vi "GearGroup.vi"(6 "Line Border":cluster{"Top":dbl, "Bottom":dbl}={"Top"=6.0, "Bottom"=1.0}, 8 "Padding for Rectangle":dbl=5.0 format="%#_13g", 9 "Score Cutoff":dbl=3.0, 10 "Sorted Data":dbl[][](array[numeric])) -> (0 "Rect":T1, 1 "Line":T1, 2 "Score":dbl, 3 "Center":cluster{"X":dbl, "Y":dbl})   [LabVIEW 2016]
panel:
  out "Grouping Scores":T2(array[cluster])
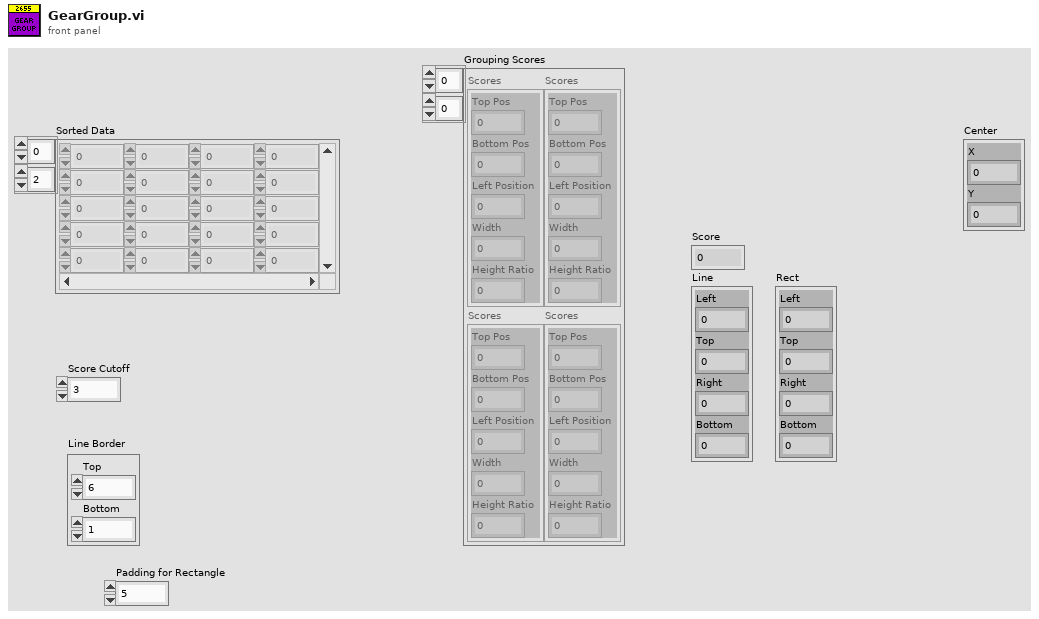
[diagram p1: front panel]
types:
  T1 = cluster{"Left":dbl, "Top":dbl, "Right":dbl, "Bottom":dbl}
  T2 = cluster{"Top Pos":dbl, "Bottom Pos":dbl, "Left Position":dbl, "Width":dbl, "Height Ratio":dbl}[][]
  T3 = cluster{"Top Position":dbl, "Bottom Position":dbl, "Top Gap":dbl, "Width":dbl, "Height Ratio":dbl}
  T4 = cluster{"Left":dbl, "Numeric":dbl, "Right":dbl, "Numeric":dbl}
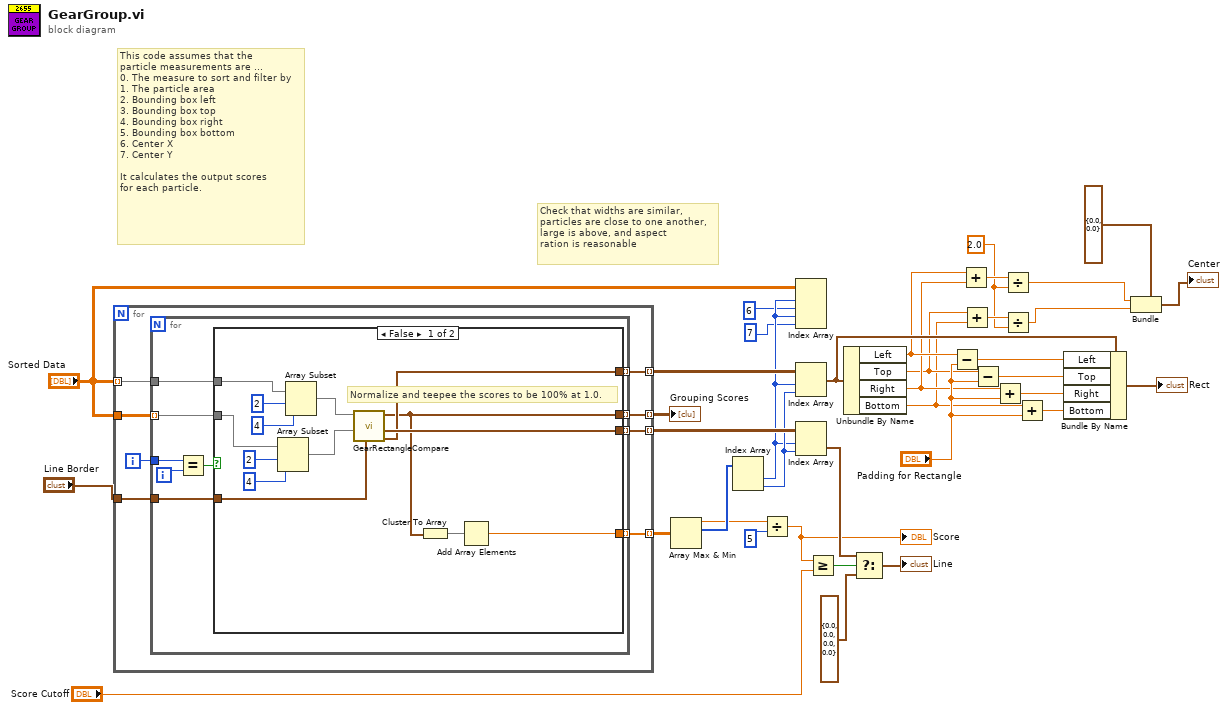
[diagram p0: block diagram]
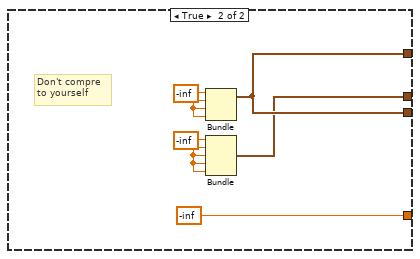
[diagram p2: hidden frame]
diagram:
  w3 = 2.0 ("y")
  # "Check that widths are similar,\nparticles are close to one another,\nlarge is above, and aspect\nration is reasonable"
  # "This code assumes that the\nparticle measurements are ...\n0. The measure to sort and filter by\n1. The particle area\n2. Bounding box left\n3. Bounding box top\n4. Bounding box right\n5. Bounding box bottom\n6. Center X\n7. Center Y\n\nIt calculates the output scores\nfor each particle."
  n1 = for {
    tunnel: "Sorted Data" -> [w45] mode=indexing
    tunnel: "Sorted Data" -> [w44]
    tunnel: [w43] -> w37 mode=indexing
    tunnel: [w41] -> w36 mode=indexing
    tunnel: [w40] -> w33 mode=indexing
    tunnel: [w39] -> w29 mode=indexing
    tunnel: "Line Border" -> [w38]
    i -> [w42]
    n2 = for {
      tunnel: w45 -> [w55]
      tunnel: w44 -> [w53] mode=indexing
      tunnel: [w52] -> w43 mode=indexing
      tunnel: w42 -> [w51]
      tunnel: [w49] -> w41 mode=indexing
      tunnel: [w48] -> w40 mode=indexing
      tunnel: [w47] -> w39 mode=indexing
      tunnel: w38 -> [w46]
      i -> [w50]
      n3 = Equal?(x=w51, y=w50) -> (x = y?=w54:bool)
      n4 = case shown="False" w54 {
        tunnel: w55 -> [w67 _]
        tunnel: w53 -> [w64 _]
        tunnel: [w58 w70] -> w52
        tunnel: [w62 -inf] -> w49
        tunnel: [w60 w73] -> w48
        tunnel: [w59 w73] -> w47
        tunnel: w46 -> [w56 _]
        frame False {
          # "Normalize and teepee the scores to be 100% at 1.0."
          n5 = Array Subset(array=w64, index=2, length=4) -> (w61:dbl[])
          n6 = Array Subset(array=w67, index=2, length=4) -> (w57:dbl[])
          n7 = call "GearRectangleCompare.vi"("Line Border"=w56, "Second"=w61, "First"=w57) -> ("Rect"=w59:T1, "Line"=w60:T1, "Scores"=w58:T3)  [unwired: 6 in]
          n8 = Cluster To Array(cluster=w58) -> (array=w63:dbl[])
          n9 = Add Array Elements(numeric array=w63) -> (sum=w62:dbl)
        }
        frame True {
          w71 = -inf
          w72 = -inf
          # "Don't compre\nto yourself"
          n10 = Bundle(w72, w72, w72, w72) -> (w73:cluster{dbl, dbl, dbl, dbl})  [unwired: 1 in]
          n11 = Bundle(w71, w71, w71, w71, w71) -> (w70:cluster{dbl, dbl, dbl, dbl, dbl})  [unwired: 1 in]
        }
      }
    }
  }
  "Grouping Scores" <- w37
  n12 = Array Max & Min(array=w36) -> (max value=w22:dbl, max index (indices)=w23:i32[])  [unwired: 2 out]
  n13 = Index Array(array=w23) -> (element #1=w26:i32, element #2=w28:i32)  [unwired: 2 in]
  n14 = Divide(x=w22, y=5 ("length")) -> (x/y=w21:dbl)
  "Score" <- w21
  n15 = Index Array(array="Sorted Data", index (row) #1=w26, index (col) #1=6 ("index"), index (row) #2=w26, index (col) #2=7 ("index")) -> ()  [unwired: 2 out]
  n16 = Index Array(array=w29, index (row)=w26, index (col)=w28) -> (element=w18:T1)
  n17 = Index Array(array=w33, index (row)=w26, index (col)=w28) -> (element=w32:T1)
  n18 = Greater Or Equal?(x=w21, y="Score Cutoff") -> (x >= y?=w35:bool)
  n19 = Unbundle By Name(w18) -> ("Left"=w10:dbl, "Top"=w6:dbl, "Right"=w9:dbl, "Bottom"=w5:dbl)
  n20 = Select(t=w32, s=w35, f=cluster{dbl, "Numeric":dbl, dbl, "Numeric":dbl} {0.0, "Numeric"=0.0, 0.0, "Numeric"=0.0}) -> (s? t:f=→"Line":T4)
  n21 = Subtract(x=w10, y="Padding for Rectangle") -> (x-y=w14:dbl)
  n22 = Add(x=w10, y=w9) -> (x+y=w8:dbl)
  n23 = Add(x=w6, y=w5) -> (x+y=w4:dbl)
  n24 = Subtract(x=w6, y="Padding for Rectangle") -> (x-y=w15:dbl)
  n25 = Add(x=w9, y="Padding for Rectangle") -> (x+y=w16:dbl)
  n26 = Divide(x=w8, y=w3) -> (x/y=w7:dbl)
  n27 = Divide(x=w4, y=w3) -> (x/y=w2:dbl)
  n28 = Add(x=w5, y="Padding for Rectangle") -> (x+y=w17:dbl)
  n29 = Bundle By Name(cluster=w18, "Left"=w14, "Top"=w15, "Right"=w16, "Bottom"=w17) -> (→"Rect":T1)
  n30 = Bundle(cluster=cluster{"X":dbl, "Y":dbl} {"X"=0.0, "Y"=0.0}, "X"=w7, "Y"=w2) -> (→"Center":cluster{"X":dbl, "Y":dbl})
